vi "Main.vi"(11 "Module Admin":refnum<class "Delacor_lib_QMH_Cloneable Module Admin.lvclass">) -> ()   [LabVIEW 2025, in "Sequencer.lvlib"]
doc: "This template is based off of the Queued Message Handler design pattern and the Queued Message Handler project template that ships with LabVIEW.\n\nThe main difference is that the queue is private to this module and communication between modules is performed via Broadcast and Request events.\n\nRequest events are wrapped in public API methods and are handled in the Event Handling Loop (EHL) of this VI. Any module can register for Broadcast events sent by this module. The EHL generates messages based on user interface actions.\n\nThe Message Handling Loop (MHL) processes messages generated by the EHL, or by other messages. The messages are string values, so new messages can be added easily to the Message Cases case structure in the MHL. Each message cluster can also provide an optional value for Message Data, which is a variant that can be converted to whatever message-specific data is required.\n_____\nBased on DQMH Dev Tools: Project Template 7.1.2.1547."
uses:
  Sequencer.lvlib
  <vilib>/Delacor/Delacor QMH/Libraries/Cloneable Module Admin_class/Delacor_lib_QMH_Cloneable Module Admin.lvclass
  C:/Program Files/National Instruments/LabVIEW 2025/vi.lib/Delacor/Delacor QMH/Libraries/Module Admin_class/Delacor_lib_QMH_Module Admin.lvclass
  Module Data--cluster.ctl
  <vilib>/Delacor/Delacor QMH/Libraries/Message Queue_class/Delacor_lib_QMH_Message Queue.lvclass/Delacor_lib_QMH_Message Queue.ctl
  <vilib>/Delacor/Delacor QMH/Libraries/Cloneable Module Admin_class/Delacor_lib_QMH_Cloneable Module Admin.lvclass/Delacor_lib_QMH_Cloneable Module Admin.ctl
  Stop Argument--cluster.ctl
  <vilib>/Delacor/Delacor QMH/Libraries/Module Admin_class/Delacor_lib_QMH_Module Admin.lvclass/Delacor_lib_QMH_Module Admin.ctl
  <vilib>/Utility/miscctls.llb/LVPointTypeDef.ctl
  <vilib>/Delacor/Delacor QMH/Libraries/Message Queue_class/Delacor_lib_QMH_Enqueue Message (Single).vi
  <vilib>/Delacor/Delacor QMH/Libraries/Cloneable Module Admin_class/Delacor_lib_QMH_Get Module ID.vi
  <vilib>/Delacor/Delacor QMH/Libraries/Module Admin_class/Delacor_lib_QMH_Get External Launch.vi
  <vilib>/Delacor/Delacor QMH/Libraries/Message Queue_class/Delacor_lib_QMH_Message Queue.lvclass
panel:
  out "error out":errorcluster
  out "Status":string
  in  "Simulate EHL Error":bool
  in  "Simulate MHL Error":bool
  # "Other processes communicate with this Module via its Public API (wrappers for its Request Events).\n\nThis Module communicates with other processes via its Broadcast Events.\nAny process that wants to receive these messages can register for this module's Broadcast events."
  # "This template is for the DQMH framework. See the block diagram for more information on how to use this template."
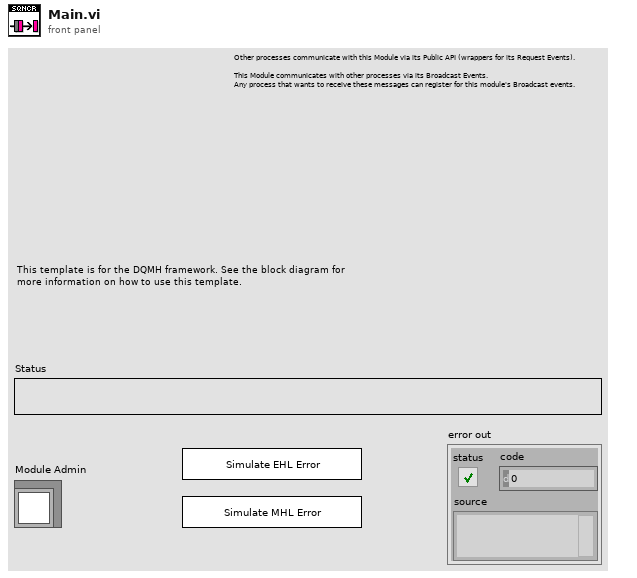
[diagram p1: front panel]
types:
  T1 = typedef "Sequencer.lvlib/Request Events--cluster.ctl" = cluster{"Stop Module":refnum<user-event>, "Show Panel":refnum<user-event>, "Hide Panel":refnum<user-event>, "Show Diagram":refnum<user-event>, "Get Module Execution Status":refnum<user-event>}
  T2 = typedef "Sequencer.lvlib/Module Data--cluster.ctl" = cluster{"Status":string}
  T3 = enum32{"invalid lock state", "Not Locked", "Locked (No Password)", "Password-protected"}
  T4 = typedef "Sequencer.lvlib/Stop Argument--cluster.ctl" = cluster{"Module ID":i32, "Origin":string, "Exit via Stop Module Req?":bool, "Wait for Module to stop?":bool}
  T5 = typedef "LVPointTypeDef.ctl" = cluster{"Horizontal":i16, "Vertical":i16}
  T6 = enum32{"Invalid", "Standard", "Closed", "Hidden", "Minimized", "Maximized"}
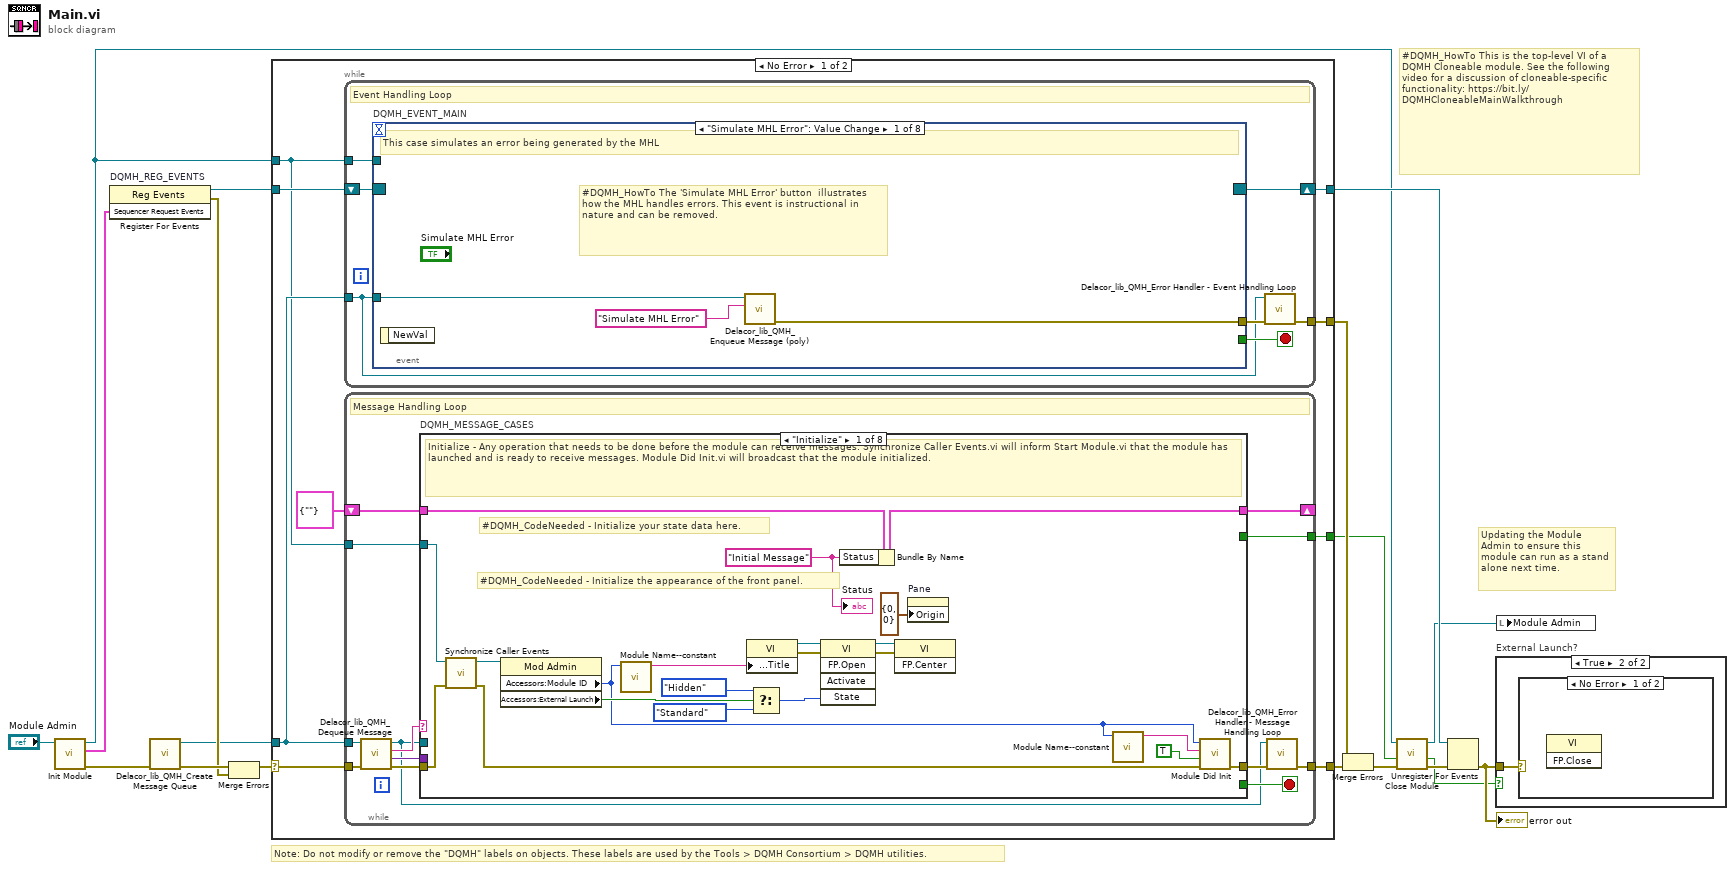
[diagram p0: block diagram]
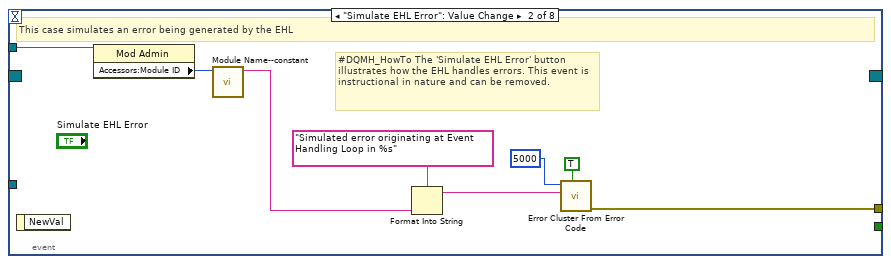
[diagram p2: hidden frame]
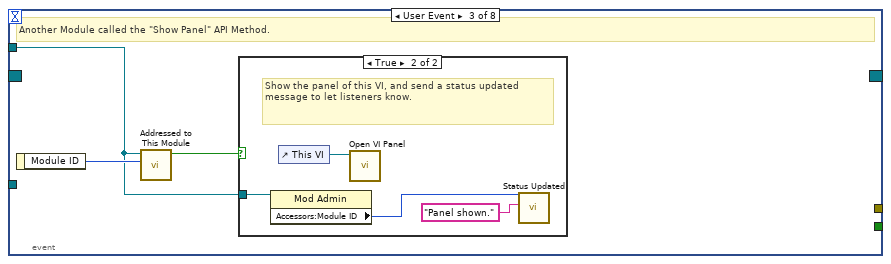
[diagram p3: hidden frame]
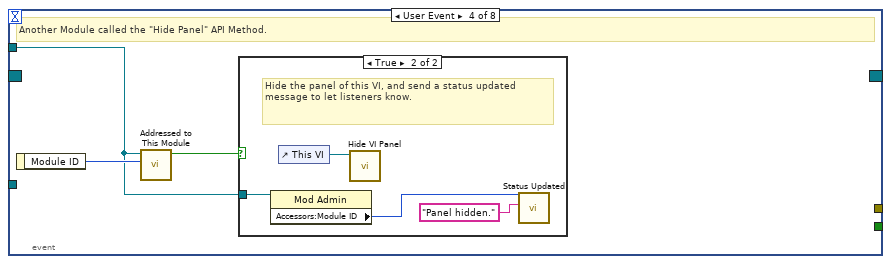
[diagram p5: hidden frame]
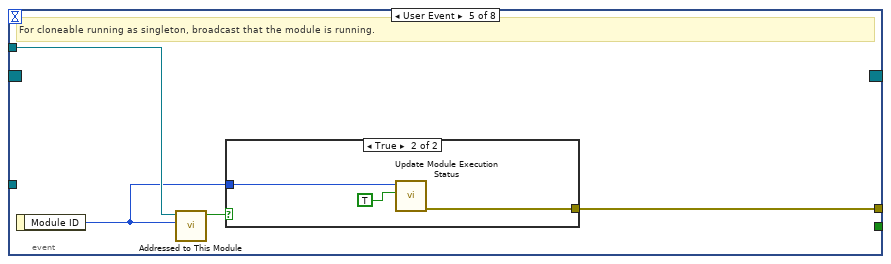
[diagram p7: hidden frame]
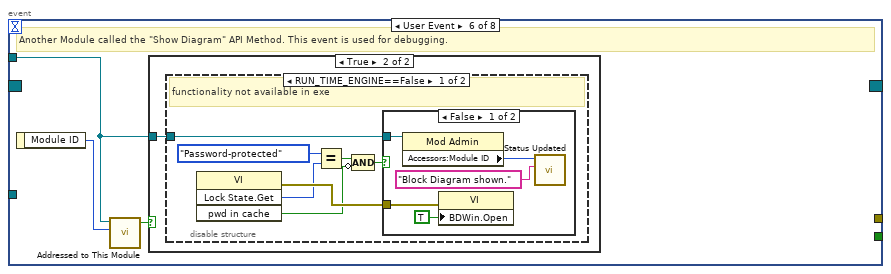
[diagram p9: hidden frame]
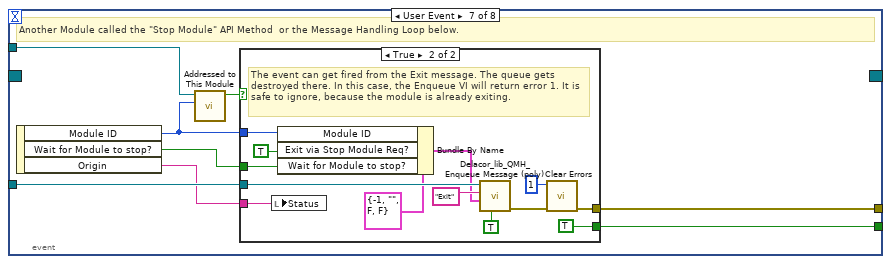
[diagram p13: hidden frame]
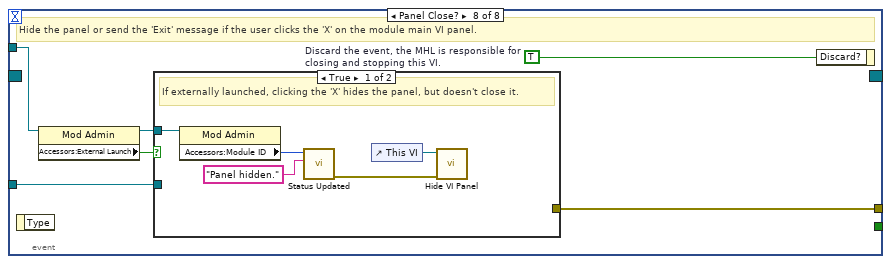
[diagram p15: hidden frame]
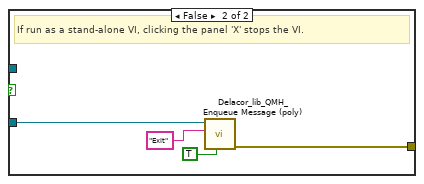
[diagram p16: hidden frame]
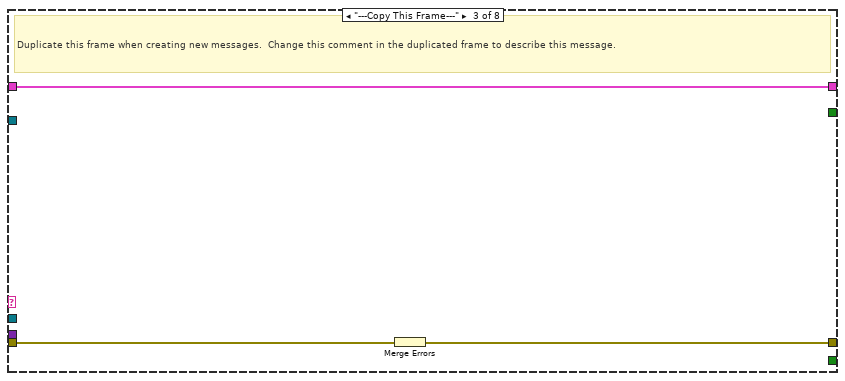
[diagram p18: hidden frame]
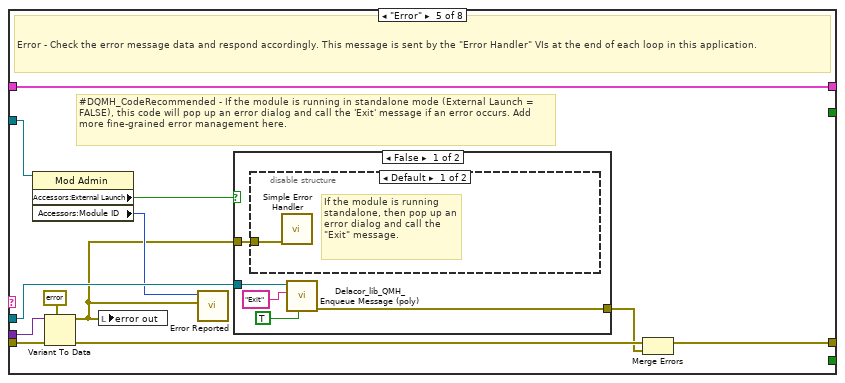
[diagram p20: hidden frame]
diagram:
  # "#DQMH_HowTo This is the top-level VI of a DQMH Cloneable module. See the following video for a discussion of cloneable-specific functionality: https://bit.ly/DQMHCloneableMainWalkthrough"
  # "Note: Do not modify or remove the \"DQMH\" labels on objects. These labels are used by the Tools > DQMH Consortium > DQMH utilities."
  # "Updating the Module Admin to ensure this module can run as a stand alone next time."
  n1 = call "Init Module.vi"("Cloneable Module Admin in"="Module Admin") -> ("error out"=w15:errorcluster, "Sequencer Request Events"=w7:T1, "Cloneable Module Admin out"=w4:refnum<class "Delacor_lib_QMH_Cloneable Module Admin.lvclass">)  [unwired: 8 in]
  n2 = register-events "DQMH_REG_EVENTS"(w7) -> (reference out=w8:refnum<event-registration>, error out=w10:errorcluster)  [unwired: 2 in]
  n3 = call <vilib>:"Delacor_lib_QMH_Create Message Queue.vi"("error in"=w15) -> ("error out"=w12:errorcluster, "Message Queue"=w6:refnum<class "Delacor_lib_QMH_Message Queue.lvclass">)  [unwired: 9 in]
  n4 = Merge Errors(w12, w10) -> (w11:errorcluster)
  n5 = case shown="No Error" w11 {
    selector: w11 -> [w25 w227]
    tunnel: [w27 w226] -> w16
    tunnel: [w24 w225] -> w9
    tunnel: w8 -> [w22 w225]
    tunnel: w6 -> [w21 w218]
    tunnel: [w26 _] -> w17
    tunnel: w4 -> [w20 w221]
    tunnel: [w19 _] -> w2
    frame No Error {
      n6 = while {
        tunnel: w21 -> [w28]
        shift-right: [w31] -> w24
        shift-left: w22 -> [w32]
        tunnel: [w33] -> w26
        tunnel: w20 -> [w29]
        stop <- w30 stop-if-true
        # "Event Handling Loop"
        n7 = event "DQMH_EVENT_MAIN" shown="[0] \"Simulate MHL Error\": Value Change" {
          selector: w32 -> [_ _ _ _ _ _ _ _]
          dyn-events: [_ _ _ _ _ _ _ _] -> w31
          timeout: _ -> [_ _ _ _ _ _ _ _]
          tunnel: [_ _ _ _ _ _ w86 _] -> w30
          tunnel: w28 -> [w36 _ _ _ _ _ w89 w106]
          tunnel: [w37 w45 _ _ w63 _ w90 w109] -> w34
          tunnel: w29 -> [_ w44 w46 w53 w61 w67 w88 w107]
          event "Simulate MHL Error": Value Change {
            # "#DQMH_HowTo The 'Simulate MHL Error' button  illustrates how the MHL handles errors. This event is instructional in nature and can be removed."
            # "This case simulates an error being generated by the MHL"
            n8 = event-data() -> ()  [unwired: 1 in, 1 out]
            n9 = call-poly <vilib>:"Delacor_lib_QMH_Enqueue Message (poly).vi"("Message"="Simulate MHL Error", "Message Queue in"=w36) -> ("error out"=w37:errorcluster)  [unwired: 8 in, 1 out]
          }
          event "Simulate EHL Error": Value Change {
            # "#DQMH_HowTo The 'Simulate EHL Error' button  illustrates how the EHL handles errors. This event is instructional in nature and can be removed."
            # "This case simulates an error being generated by the EHL"
            n10 = event-data() -> ()  [unwired: 1 in, 1 out]
            n11 = property on="Property Node" class="Mod Admin"(reference=w44) -> ("Accessors:Module ID"=w43:i32)  [unwired: 1 in, 2 out]
            n12 = call "Module Name--constant.vi"("Module ID"=w43) -> ("Module Name"=w38:string)  [unwired: 10 in]
            n13 = Format Into String(format string="Simulated error originating at Event Handling Loop in %s", w38) -> (resulting string=w41:string)  [unwired: 2 in, 1 out]
            n14 = call <vilib>:"Error Cluster From Error Code.vi"("show call chain? (False)"=TRUE, "error message (\"\")"=w41, "error code (0)"=5000) -> ("error out"=w45:errorcluster)  [unwired: 6 in]
          }
          event User Event {
            # "Another Module called the \"Show Panel\" API Method."
            n15 = event-data() -> ("Module ID"=w47:i32)  [unwired: 1 in]
            n16 = call "Addressed to This Module.vi"("Module ID from Argument"=w47, "Module Admin"=w46) -> ("Addressed to this instance?"=w48:bool)  [unwired: 8 in, 1 out]
            n17 = case shown="True" w48 {
              tunnel: w46 -> [_ w50]
              frame False {
              }
              frame True {
                # "Show the panel of this VI, and send a status updated message to let listeners know."
                n18 = property on="Property Node" class="Mod Admin"(reference=w50) -> ("Accessors:Module ID"=w49:i32)  [unwired: 1 in, 2 out]
                n19 = control-ref of="This VI"() -> (w52:refnum<vi>)
                n20 = call "Open VI Panel.vi"("VI"=w52) -> ()  [unwired: 10 in, 1 out]
                n21 = call "Status Updated.vi"("Status"="Panel shown." ("format string"), "Module ID"=w49) -> ()  [unwired: 9 in, 1 out]
              }
            }
          }
          event User Event {
            # "Another Module called the \"Hide Panel\" API Method."
            n22 = event-data() -> ("Module ID"=w54:i32)  [unwired: 1 in]
            n23 = call "Addressed to This Module.vi"("Module ID from Argument"=w54, "Module Admin"=w53) -> ("Addressed to this instance?"=w55:bool)  [unwired: 8 in, 1 out]
            n24 = case shown="True" w55 {
              tunnel: w53 -> [_ w57]
              frame False {
              }
              frame True {
                # "Hide the panel of this VI, and send a status updated message to let listeners know."
                n25 = property on="Property Node" class="Mod Admin"(reference=w57) -> ("Accessors:Module ID"=w56:i32)  [unwired: 1 in, 2 out]
                n26 = control-ref of="This VI"() -> (w59:refnum<vi>)
                n27 = call "Hide VI Panel.vi"("VI"=w59) -> ()  [unwired: 10 in, 1 out]
                n28 = call "Status Updated.vi"("Status"="Panel hidden." ("format string"), "Module ID"=w56) -> ()  [unwired: 9 in, 1 out]
              }
            }
          }
          event User Event {
            # "For cloneable running as singleton, broadcast that the module is running."
            n29 = event-data() -> ("Module ID"=w60:i32)  [unwired: 1 in]
            n30 = call "Addressed to This Module.vi"("Module ID from Argument"=w60, "Module Admin"=w61) -> ("Addressed to this instance?"=w62:bool)  [unwired: 8 in, 1 out]
            n31 = case shown="True" w62 {
              tunnel: [_ w66] -> w63
              tunnel: w60 -> [_ w65]
              frame False {
              }
              frame True {
                n32 = call "Update Module Execution Status.vi"("Running?"=TRUE, "Module ID"=w65) -> ("error out"=w66:errorcluster)  [unwired: 9 in]
              }
            }
          }
          event User Event {
            # "Another Module called the \"Show Diagram\" API Method. This event is used for debugging."
            n33 = event-data() -> ("Module ID"=w68:i32)  [unwired: 1 in]
            n34 = call "Addressed to This Module.vi"("Module ID from Argument"=w68, "Module Admin"=w67) -> ("Addressed to this instance?"=w69:bool)  [unwired: 8 in, 1 out]
            n35 = case shown="True" w69 {
              tunnel: w67 -> [_ w70]
              frame False {
              }
              frame True {
                n36 = disable-structure shown="RUN_TIME_ENGINE==False" {
                  disable-tunnel: w70 -> [w71 _]
                  frame condition #0 (active) {
                    # "functionality not available in exe"
                    n37 = invoke on="Invoke Node" class="VI" method="Lock State.Get"() -> (error out=w77:errorcluster, "Get Lock State"=w76:T3, "pwd in cache"=w73:bool)  [unwired: 4 in, 1 out]
                    n38 = Equal?(x=T3."Password-protected", y=w76) -> (x = y?=w74:bool)
                    n39 = Compound Arithmetic op=AND(w74, invert w73) -> (w72:bool)
                    n40 = case shown="False" w72 {
                      tunnel: w77 -> [w82 _]
                      tunnel: w71 -> [w79 _]
                      frame False {
                        n41 = property on="Property Node" class="Mod Admin"(reference=w79) -> ("Accessors:Module ID"=w78:i32)  [unwired: 1 in, 2 out]
                        n42 = property on="Property Node" class="VI"(error in=w82, "BDWin.Open"=TRUE ("Block Diagram Window:Open")) -> ()  [unwired: 1 in, 2 out]
                        n43 = call "Status Updated.vi"("Status"="Block Diagram shown." ("format string"), "Module ID"=w78) -> ()  [unwired: 9 in, 1 out]
                      }
                      frame True {
                        # "Password-protected VI, and the password is not in the cache. Do not show the diagram."
                      }
                    }
                  }
                  frame condition #1 {
                  }
                }
              }
            }
          }
          event User Event {
            # "Another Module called the \"Stop Module\" API Method  or the Message Handling Loop below."
            n44 = event-data() -> ("Module ID"=w84:i32, "Wait for Module to stop?"=w85:bool, "Origin"=w83:string)  [unwired: 1 in]
            n45 = call "Addressed to This Module.vi"("Module ID from Argument"=w84, "Module Admin"=w88) -> ("Addressed to this instance?"=w87:bool)  [unwired: 8 in, 1 out]
            n46 = case shown="True" w87 {
              tunnel: [_ w102] -> w90
              tunnel: w89 -> [_ w98]
              tunnel: [_ TRUE] -> w86
              tunnel: w85 -> [_ w93]
              tunnel: w84 -> [_ w95]
              tunnel: w83 -> [_ w91]
              frame False {
              }
              frame True {
                # "The event can get fired from the Exit message. The queue gets destroyed there. In this case, the Enqueue VI will return error 1. It is safe to ignore, because the module is already exiting."
                n47 = local write "Status"(w91) -> ()
                n48 = Bundle By Name(cluster=T4 {"Module ID"=-1, "Origin"="", "Exit via Stop Module Req?"=FALSE, "Wait for Module to stop?"=FALSE} ("Stop Argument"), "Module ID"=w95, "Exit via Stop Module Req?"=TRUE, "Wait for Module to stop?"=w93) -> (w92:T4)
                n49 = call-poly <vilib>:"Delacor_lib_QMH_Enqueue Message (poly).vi"("Priority Message? (F)"=TRUE, "Message Data"=w92, "Message"="Exit", "Message Queue in"=w98) -> ("error out"=w103:errorcluster)  [unwired: 6 in, 1 out]
                n50 = call <vilib>:"Clear Errors.vi"("error in (no error)"=w103, "specific error code to clear (0: all)"=1) -> ("error out"=w102:errorcluster)  [unwired: 4 in, 1 out]
              }
            }
          }
          event Panel Close? {
            w108 = TRUE  # Discard the event, the MHL is responsible for closing and stopping this VI.
            # "Hide the panel or send the 'Exit' message if the user clicks the 'X' on the module main VI panel."
            n51 = event-data() -> ()  [unwired: 1 in, 1 out]
            n52 = property on="Property Node" class="Mod Admin"(reference=w107) -> (reference out=w104:refnum<class "Delacor_lib_QMH_Cloneable Module Admin.lvclass">, "Accessors:External Launch"=w105:bool)  [unwired: 1 in, 1 out]
            n53 = case shown="True" w105 {
              tunnel: w106 -> [_ w117]
              tunnel: [_ w118] -> w109
              tunnel: w104 -> [w112 _]
              frame True {
                # "If externally launched, clicking the 'X' hides the panel, but doesn't close it."
                n54 = property on="Property Node" class="Mod Admin"(reference=w112) -> ("Accessors:Module ID"=w111:i32)  [unwired: 1 in, 2 out]
                n55 = call "Status Updated.vi"("Status"="Panel hidden." ("format string"), "Module ID"=w111) -> ("error out"=w110:errorcluster)  [unwired: 9 in]
                n56 = control-ref of="This VI"() -> (w114:refnum<vi>)
                n57 = call "Hide VI Panel.vi"("error in"=w110, "VI"=w114) -> ()  [unwired: 9 in, 1 out]
              }
              frame False {
                # "If run as a stand-alone VI, clicking the panel 'X' stops the VI."
                n58 = call-poly <vilib>:"Delacor_lib_QMH_Enqueue Message (poly).vi"("Priority Message? (F)"=TRUE, "Message"="Exit", "Message Queue in"=w117) -> ("error out"=w118:errorcluster)  [unwired: 7 in, 1 out]
              }
            }
            n59 = event-data ("Event Filter Node")("Discard?"=w108) -> ()  [unwired: 1 in, 1 out]
          }
        }
        n60 = call-dynamic "Delacor_lib_QMH_Error Handler - Event Handling Loop.vi"("error in"=w34, "Message Queue in"=w28) -> ("dup error in"=w33:errorcluster)  [unwired: 8 in, 1 out]
      }
      n61 = while {
        tunnel: w21 -> [w119]
        shift-right: [w126] -> _
        shift-left: T2 {"Status"=""} ("Data Cluster") -> [w127]
        tunnel: w25 -> [w130]
        tunnel: [w128] -> w27
        tunnel: w20 -> [w121]
        tunnel: [w120] -> w19
        stop <- w125 stop-if-true
        # "Message Handling Loop"
        n62 = call-dynamic "Delacor_lib_QMH_Dequeue Message.vi"("error in"=w130, "Message Queue in"=w119) -> ("error out"=w129:errorcluster, "Message Data"=w123:variant, "Message"=w124:string, "Message Queue out"=w122:refnum<class "Delacor_lib_QMH_Message Queue.lvclass">)  [unwired: 6 in]
        n63 = case "DQMH_MESSAGE_CASES" shown="\"Initialize\"" w124 {
          selector: w124 -> [_ _ _ _ _ _ _ w207]
          tunnel: w122 -> [_ _ _ _ w162 _ w199 _]
          tunnel: w129 -> [w150 w154 w157 w159 w171 w188 w205 w216]
          tunnel: [w148 w154 w156 w159 w167 w187 w200 w217] -> w131
          tunnel: w127 -> [w141 w153 w155 w158 w166 w185 w198 w214]
          tunnel: [w140 w153 w155 w158 w166 w185 w198 w214] -> w126
          tunnel: [_ _ _ _ _ _ w197 _] -> w125
          tunnel: w123 -> [_ _ _ _ w165 _ w195 _]
          tunnel: w121 -> [w136 _ _ _ w164 w183 w190 w213]
          tunnel: [_ _ _ _ _ _ w193 _] -> w120
          frame "Initialize" {
            w133 = "Initial Message" ("Initial Message")
            # "#DQMH_CodeNeeded - Initialize the appearance of the front panel."
            # "#DQMH_CodeNeeded - Initialize your state data here."
            # "Initialize - Any operation that needs to be done before the module can receive messages. Synchronize Caller Events.vi will inform Start Module.vi that the module has launched and is ready to receive messages. Module Did Init.vi will broadcast that the module initialized."
            n64 = call "Synchronize Caller Events.vi"("error in"=w150, "Module Admin"=w136) -> ("error out"=w149:errorcluster, "Module Admin out"=w135:refnum<class "Delacor_lib_QMH_Cloneable Module Admin.lvclass">)  [unwired: 8 in]
            n65 = property on="Property Node" class="Mod Admin"(reference=w135) -> ("Accessors:Module ID"=w132:i32, "Accessors:External Launch"=w137:bool)  [unwired: 1 in, 2 out]
            n66 = call "Module Name--constant.vi"("Module ID"=w132) -> ("Module Name"=w145:string)  [unwired: 10 in]
            n67 = property on="Property Node" class="VI"("Front Panel.Title"=w145) -> (reference out=w147:refnum<vi>, error out=w152:errorcluster)  [unwired: 2 in]
            n68 = Select(t=T6."Hidden" ("State"), s=w137, f=T6."Standard" ("State")) -> (s? t:f=w142:T6)
            n69 = invoke on="Invoke Node" class="VI" method="FP.Open"(reference=w147, error in=w152, "State"=w142) -> (reference out=w146:refnum<vi>, error out=w151:errorcluster)  [unwired: 2 in, 3 out]
            n70 = Bundle By Name(cluster=w141, "Status"=w133) -> (w140:T2)
            n71 = invoke on="Invoke Node" class="VI" method="FP.Center"(reference=w146, error in=w151) -> ()  [unwired: 1 in, 3 out]
            n72 = property on="Pane" class="Pane"("Origin"=T5 {"Horizontal"=0, "Vertical"=0}) -> ()  [unwired: 2 in, 2 out]
            n73 = call "Module Name--constant.vi"("Module ID"=w132) -> ("Module Name"=w138:string)  [unwired: 10 in]
            n74 = call "Module Did Init.vi"("error in"=w149, "Initialized?"=TRUE, "Origin"=w138, "Module ID"=w132) -> ("error out"=w148:errorcluster)  [unwired: 7 in]
            "Status" <- w133
          }
          frame "---Module Specific---" {
            # "Separator -- The following cases handle messages specific to this Module."
          }
          frame "---Copy This Frame---" {
            # "Duplicate this frame when creating new messages.  Change this comment in the duplicated frame to describe this message."
            n75 = Merge Errors(w157) -> (w156:errorcluster)
          }
          frame "---Exit and Error Handling---" {
            # "Separator - the following cases handle errors and exit messages."
          }
          frame "Error" {
            # "#DQMH_CodeRecommended - If the module is running in standalone mode (External Launch = FALSE), this code will pop up an error dialog and call the 'Exit' message if an error occurs. Add more fine-grained error management here."
            # "Error - Check the error message data and respond accordingly. This message is sent by the \"Error Handler\" VIs at the end of each loop in this application."
            n76 = property on="Property Node" class="Mod Admin"(reference=w164) -> ("Accessors:External Launch"=w163:bool, "Accessors:Module ID"=w161:i32)  [unwired: 1 in, 2 out]
            n77 = Variant To Data(error in=w171, type=errorcluster {"status"=FALSE, "code"=0, "source"=""} ("error constant"), Variant=w165) -> (data=w160:errorcluster, error out=w169:errorcluster)
            n78 = local write "error out"(w160) -> ()
            n79 = call "Error Reported.vi"("Error"=w160, "Module ID"=w161) -> ()  [unwired: 9 in, 1 out]
            n80 = case shown="False" w163 {
              tunnel: [w176 _] -> w168
              tunnel: w162 -> [w174 _]
              tunnel: w160 -> [w175 _]
              frame False {
                n81 = disable-structure shown="Default" {
                  disable-tunnel: w175 -> [w177 _]
                  frame condition #0 (active) {
                    # "If the module is running standalone, then pop up an error dialog and call the \"Exit\" message."
                    n82 = call <vilib>:"Simple Error Handler.vi"("error in (no error)"=w177) -> ()  [unwired: 4 in, 5 out]
                  }
                  frame condition #1 {
                    # "To prevent the Simple Error Handler VI from being loaded (e.g. when deploying to a Real-Time target), add the Conditional Disable Symbol \"DQMH_Disable_SEH\" to your project and set it to TRUE."
                  }
                }
                n83 = call-poly <vilib>:"Delacor_lib_QMH_Enqueue Message (poly).vi"("Priority Message? (F)"=TRUE, "Message"="Exit", "Message Queue in"=w174) -> ("error out"=w176:errorcluster)  [unwired: 7 in, 1 out]
              }
              frame True {
                # "If the module was launched externally, calling the Error Reported broadcast VI is the only action performed by the \"Error\" message. The module's caller can then process the error appropriately."
              }
            }
            n84 = Merge Errors(w169, w168) -> (w167:errorcluster)
          }
          frame "Simulate MHL Error" {
            # "#DQMH_HowTo The 'Simulate MHL Error' button  illustrates how the MHL handles errors. This event is instructional in nature and can be removed."
            # "Simulate an error occurring at the MHL"
            n85 = property on="Property Node" class="Mod Admin"(reference=w183) -> ("Accessors:Module ID"=w184:i32)  [unwired: 1 in, 2 out]
            n86 = call "Module Name--constant.vi"("Module ID"=w184) -> ("Module Name"=w179:string)  [unwired: 10 in]
            n87 = Format Into String(format string="Simulated error originating at Message Handling Loop in %s", w179) -> (resulting string=w180:string)  [unwired: 2 in, 1 out]
            n88 = call <vilib>:"Error Cluster From Error Code.vi"("show call chain? (False)"=TRUE, "error message (\"\")"=w180, "error code (0)"=5001) -> ("error out"=w186:errorcluster)  [unwired: 6 in]
            n89 = Merge Errors(w188, w186) -> (w187:errorcluster)
          }
          frame "Exit" {
            w196 = 91  # 91: not all Exit messages will have an argument
            w197 = TRUE  # Stop the VI
            # "Release the message queue reference"
            # "#DQMH_CodeNeeded - Add any required cleanup code here."
            # "Exit - Exit the application."
            n90 = Variant To Data(error in=w205, type=T4 {"Module ID"=-1, "Origin"="", "Exit via Stop Module Req?"=FALSE, "Wait for Module to stop?"=FALSE} ("Stop Argument"), Variant=w195) -> (data=w192:T4, error out=w201:errorcluster)
            n91 = call <vilib>:"Clear Errors.vi"("error in (no error)"=w201, "specific error code to clear (0: all)"=w196) -> ("error out"=w204:errorcluster)  [unwired: 4 in, 1 out]
            n92 = property on="Property Node" class="Mod Admin"(reference=w190) -> ("Accessors:Module ID"=w189:i32)  [unwired: 1 in, 2 out]
            n93 = control-ref of="This VI"() -> (w191:refnum<vi>)
            n94 = call-dynamic "Delacor_lib_QMH_Release Message Queue.vi"("error in"=w204, "Message Queue"=w199) -> ("error out"=w203:errorcluster)  [unwired: 9 in]
            n95 = call "Handle Exit.vi"("Stop Argument"=w192, "Module Admin in"=w190, "VI reference"=w191) -> ("error out"=w202:errorcluster, "Wait for Stop?"=w193:bool)  [unwired: 7 in]
            n96 = Merge Errors(w203, w202) -> (w200:errorcluster)
            n97 = call "Error Reported.vi"("Error"=w200, "Module ID"=w189) -> ()  [unwired: 9 in, 1 out]
          }
          frame Default {
            # "'Default' case only runs if there is a message that isn't defined in any of the other cases.  Output a programming error."
            n98 = property on="Property Node" class="Mod Admin"(reference=w213) -> ("Accessors:Module ID"=w212:i32)  [unwired: 1 in, 2 out]
            n99 = call "Module Name--constant.vi"("Module ID"=w212) -> ("Module Name"=w206:string)  [unwired: 10 in]
            n100 = Format Into String(format string="The invalid message string \"%s\" was received in the Message Handling Loop for module \"%s\".", w207, w206) -> (resulting string=w209:string)  [unwired: 2 in, 1 out]
            n101 = call <vilib>:"Error Cluster From Error Code.vi"("show call chain? (False)"=TRUE, "error message (\"\")"=w209, "error code (0)"=1) -> ("error out"=w215:errorcluster)  [unwired: 6 in]
            n102 = Merge Errors(w216, w215) -> (w217:errorcluster)
          }
        }
        n103 = call-dynamic "Delacor_lib_QMH_Error Handler - Message Handling Loop.vi"("error in"=w131, "Message Queue in"=w122) -> ("dup error in"=w128:errorcluster)  [unwired: 8 in, 1 out]
      }
    }
    frame Error {
      n104 = call "Synchronize Caller Events.vi"("Module Admin"=w221) -> ("Module Admin out"=w220:refnum<class "Delacor_lib_QMH_Cloneable Module Admin.lvclass">)  [unwired: 9 in, 1 out]
      n105 = property on="Property Node" class="Mod Admin"(reference=w220) -> ("Accessors:Module ID"=w219:i32)  [unwired: 1 in, 2 out]
      n106 = call-dynamic "Delacor_lib_QMH_Release Message Queue.vi"("error in"=w227, "Message Queue"=w218) -> ("error out"=w226:errorcluster)  [unwired: 9 in]
      n107 = call "Module Name--constant.vi"("Module ID"=w219) -> ("Module Name"=w224:string)  [unwired: 10 in]
      n108 = Format Into String(format string="An error occurred during initialization. %s is no longer running.", w224) -> (resulting string=w222:string)  [unwired: 2 in, 1 out]
      n109 = call "Error Reported.vi"("Additional Information"=w222, "Error"=w226, "Module ID"=w219) -> ()  [unwired: 8 in, 1 out]
    }
  }
  n110 = Merge Errors(w17, w16) -> (w18:errorcluster)
  n111 = call "Close Module.vi"("error in"=w18, "Wait for stop?"=w2, "Module Admin in"=w4) -> ("error out"=w14:errorcluster, "External Launch"=w1:bool, "Module Admin out"=w3:refnum<class "Delacor_lib_QMH_Cloneable Module Admin.lvclass">)  [unwired: 6 in]
  n112 = Unregister For Events(event registration refnum=w9, error in=w14) -> (error out=w13:errorcluster)
  "error out" <- w13
  n113 = case "External Launch?" shown="True" w1 {
    tunnel: w13 -> [_ w228]
    frame False {
    }
    frame True {
      n114 = case shown="No Error" w228 {
        frame No Error {
          n115 = invoke class="VI" method="FP.Close"() -> ()  [unwired: 3 in, 3 out]
        }
        frame Error {
          n116 = disable-structure shown="Default" {
            frame condition #0 (active) {
              n117 = invoke class="VI" method="FP.Open"("Activate"=TRUE ("Activate?")) -> ()  [unwired: 4 in, 5 out]
            }
            frame condition #1 {
              # "Don't show panel on error if running inside a built EXE."
            }
          }
        }
      }
    }
  }
  n118 = local write "Module Admin"(w3) -> ()
